vi "Read Heading Command Message.vi"(8 "error in (no error)":errorcluster, 11 "Heading Command Msg in":refnum<class "Heading Command Msg.lvclass">) -> (0 "error out":errorcluster, 2 "Heading Command Control":T1, 3 "Heading Command Msg out":refnum<class "Heading Command Msg.lvclass">)   [LabVIEW 2015, in "RDS Child Messages.lvlib" / "Heading Command Msg.lvclass"]
uses:
  Heading Command Msg.lvclass
  Heading Command Cntrl.ctl
  Heading Command Msg.lvclass/Heading Command Msg.ctl
  RDS Child Messages.lvlib
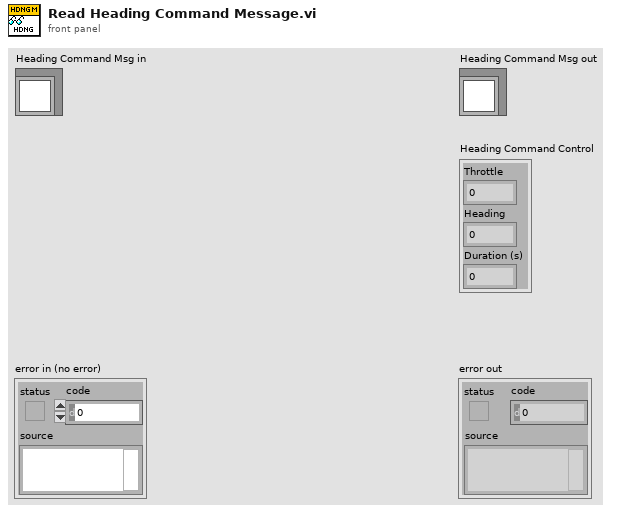
[diagram p1: front panel]
types:
  T1 = typedef "RDS Child Messages.lvlib/Heading Command Cntrl.ctl" = cluster{"Throttle":i16, "Heading":sgl, "Duration (s)":i16}
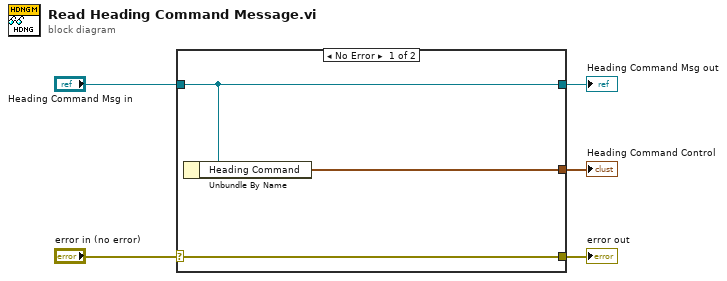
[diagram p0: block diagram]
diagram:
  n1 = case shown="No Error" "error in (no error)" {
    selector: "error in (no error)" -> [w8 w9]
    tunnel: [w8 w9] -> w4
    tunnel: [w7 w10] -> w2
    tunnel: "Heading Command Msg in" -> [w7 w10]
    tunnel: [w6 _] -> w1
    frame No Error {
      n2 = Unbundle By Name(w7) -> ("Heading Command"=w6:T1)
    }
    frame Error {
    }
  }
  "error out" <- w4
  "Heading Command Msg out" <- w2
  "Heading Command Control" <- w1
